vi "2.vi"(9 "2":dbl, 10 "Numeric":i32, 11 "Numeric 2":i32) -> (3 "Array":u32[](array[numeric]))   [LabVIEW 2016]
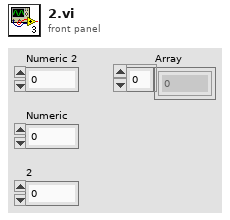
[diagram p1: front panel]
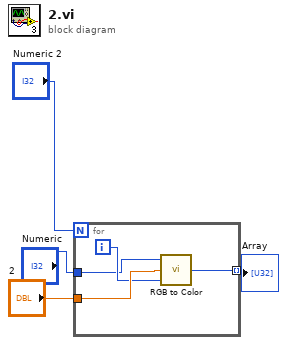
[diagram p0: block diagram]
diagram:
  n1 = for {
    N: "Numeric 2" -> [_]
    tunnel: [w8] -> w1 mode=indexing
    tunnel: "Numeric" -> [w5]
    tunnel: "2" -> [w7]
    i -> [w6]
    n2 = call <vilib>:"RGB to Color.vi"("B"=w6, "G"=w7, "R"=w5) -> ("Color"=w8:u32)
  }
  "Array" <- w1
